vi "PV Run-up time.vi"(8 "error in (no error)":errorcluster, 9 "PV Run-up time - Cluster":T1={"Parameter"=0, "Parameter\nread only<->describe"=FALSE, "Run-up time monitoring\noff     <----->     on"=TRUE, "maximum run-up\ntime [min]"=15, "speed switchpoint\n1 + 2  [%]"=80, "configuration rotation\nspeed switchpoint"=0} {"configuration rotation\nspeed switchpoint" items=["rotation speed switchpoint 1 ", "rotation speed switchpoint 1 & 2"]; "Parameter" items=["Run-up time monitoring [off/on] (004)", "run-up time [min] (700)", "speed switchpoint 1 [%] (701)", "speed switchpoint 2 [%] (719)", "configuration rotation speed switchpoint (017)"]; "speed switchpoint\n1 + 2  [%]" min=40 max=98 step=1; "maximum run-up\ntime [min]" min=1 max=120 step=1}, 10 "Adress of unit":u16=1 min=1 max=999 step=1, 11 "VISA session":refnum<visa-resource-name>) -> (0 "error out":errorcluster, 2 "response (data)":string, 3 "dup VISA session":refnum<visa-resource-name>)   [LabVIEW 2021, in "Pfeiffer Vacuum.lvlib"]
doc: "There are 5 parameters available, only one of which can be enabled at a time. \n\nRun-up time monitoring [off/on] (default) (004)\nmaximum run-up time [min] (700)\nspeed switchpoint 1 [%] (701)\nspeed switchpoint 2 [%] (719)\nconfiguration rotation speed switchpoint (017]\n\nNote: Any settings for an parameter that is not selected will be ignored. If a value is out of range, it will be changed to either the upper or the lower limit of the range."
uses:
  <instrlib>/Pfeiffer Vacuum/Pfeiffer Vacuum.lvlib
  <instrlib>/Pfeiffer Vacuum/Public/Turbopumps/PV Run-up time - Cluster.ctl
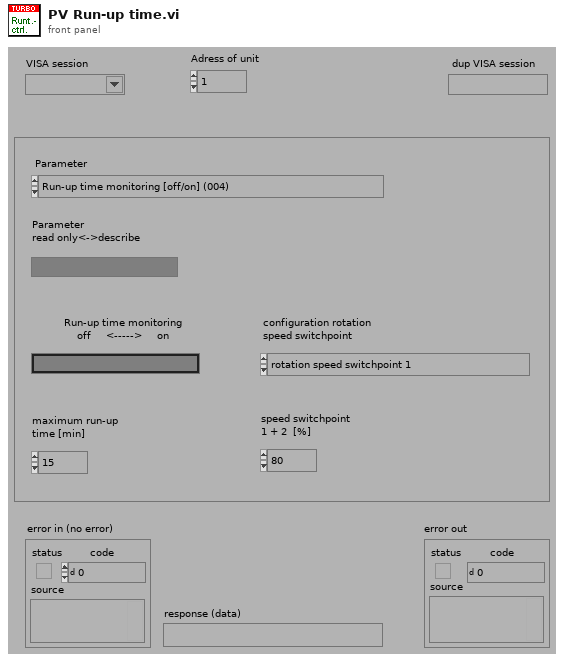
[diagram p1: front panel]
types:
  T1 = typedef "Pfeiffer Vacuum.lvlib/PV Run-up time - Cluster.ctl" = cluster{"Parameter":u16, "Parameter\nread only<->describe":bool, "Run-up time monitoring\noff     <----->     on":bool, "maximum run-up\ntime [min]":u16, "speed switchpoint\n1 + 2  [%]":u16, "configuration rotation\nspeed switchpoint":u16}
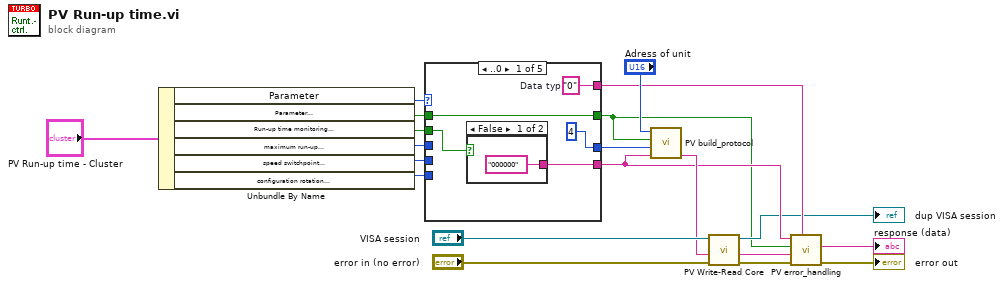
[diagram p0: block diagram]
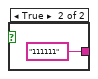
[diagram p2: hidden frame]
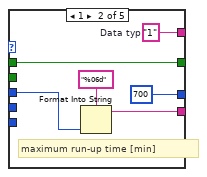
[diagram p3: hidden frame]
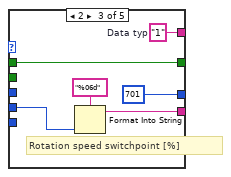
[diagram p4: hidden frame]
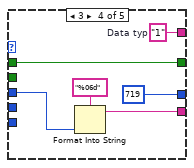
[diagram p5: hidden frame]
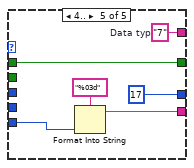
[diagram p6: hidden frame]
diagram:
  n1 = Unbundle By Name("PV Run-up time - Cluster") -> ("Parameter"=w8:u16, "Parameter\nread only<->describe"=w7:bool, "Run-up time monitoring\noff     <----->     on"=w5:bool, "maximum run-up\ntime [min]"=w4:u16, "speed switchpoint\n1 + 2  [%]"=w3:u16, "configuration rotation\nspeed switchpoint"=w1:u16)
  n2 = case shown="..0" w8 {
    tunnel: [u16 4 ("Parameter-number") u16 700 ("Parameter-number") u16 701 ("Parameter-number") u16 719 ("Parameter-number") u16 17 ("Parameter-number")] -> w19
    tunnel: [w24 w32 w38 w44 w50] -> w14
    tunnel: [w23 w30 w36 w42 w48] -> w15
    tunnel: w7 -> [w22 w29 w35 w41 w47]
    tunnel: [w22 w29 w35 w41 w47] -> w6
    tunnel: w5 -> [w21 _ _ _ _]
    tunnel: w4 -> [_ w28 _ w40 _]
    tunnel: w3 -> [_ _ w34 _ _]
    tunnel: w1 -> [_ _ _ _ w46]
    frame ..0 {
      w23 = "0"  # Data typ
      n3 = case shown="False" w21 {
        tunnel: ["000000" ("Data") "111111" ("Data")] -> w24
        frame False {
        }
        frame True {
        }
      }
    }
    frame 1 {
      w30 = "1"  # Data typ
      # "maximum run-up time [min]"
      n4 = Format Into String(format string="%06d" ("Format-String"), w28) -> (resulting string=w32:string)  [unwired: 2 in, 1 out]
    }
    frame 2 {
      w36 = "1"  # Data typ
      # "Rotation speed switchpoint [%]"
      n5 = Format Into String(format string="%06d" ("Format-String"), w34) -> (resulting string=w38:string)  [unwired: 2 in, 1 out]
    }
    frame 3 {
      w42 = "1"  # Data typ
      n6 = Format Into String(format string="%06d" ("Format-String"), w40) -> (resulting string=w44:string)  [unwired: 2 in, 1 out]
    }
    frame 4.. {
      w48 = "7"  # Data typ
      n7 = Format Into String(format string="%03d" ("Format-String"), w46) -> (resulting string=w50:string)  [unwired: 2 in, 1 out]
    }
  }
  n8 = call <instrlib>:"PV build_protocol.vi"("Data"=w14, "Parameter-number"=w19, "parameter\nread<->describe"=w6, "Adress"="Adress of unit") -> ("output"=w16:string)  [unwired: 3 in]
  n9 = call <instrlib>:"PV Write-Read Core.vi"("error in"="error in (no error)", "Write data in"=w16, "VISA session"="VISA session") -> ("error out"=w12:errorcluster, "response (data) out"=w13:string, "dup VISA session"=→"dup VISA session":refnum<visa-resource-name>)  [unwired: 2 in]
  n10 = call <instrlib>:"PV error_handling.vi"("Data Typ in"=w15, "error in"=w12, "response (data) in"=w13, "Parameter\nread only<->describe"=w6, "data in"=w14) -> ("error out"=→"error out":errorcluster, "Data out"=→"response (data)":string)  [unwired: 4 in, 1 out]
